vi "ElevatorControl.vi"(2 "Intake Active":bool, 3 "BallThereAtBottom?":bool, 4 "BallThereAtTop?":bool, 5 "WantToShoot?":bool) -> (0 "HopperWheelsOn":bool, 1 "ElevatorOn":bool)   [LabVIEW 2019]
uses:
  ArgosLib/ArgosLib.lvlib
panel:
  in  "IntakeHopperTime(ms)":u32=1000
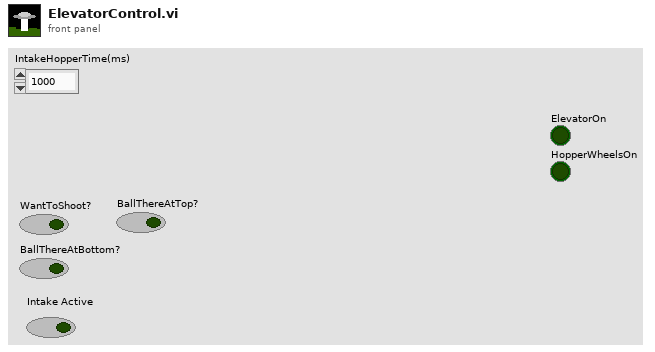
[diagram p1: front panel]
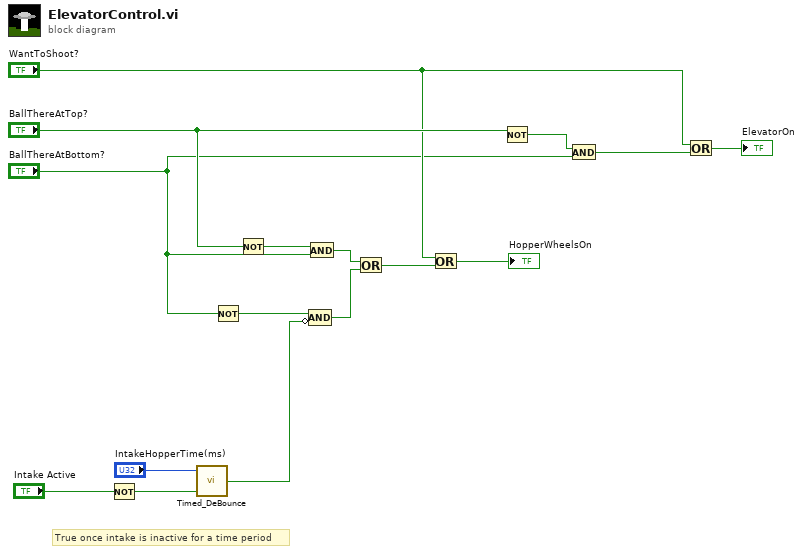
[diagram p0: block diagram]
diagram:
  # "True once intake is inactive for a time period"
  n1 = Not(x="Intake Active") -> (.not. x?=w7:bool)
  n2 = call "Timed_DeBounce.vi"("Input"=w7, "Hold Time(ms)"="IntakeHopperTime(ms)") -> ("Output"=w3:bool)  [unwired: 1 in]
  n3 = Not(x="BallThereAtBottom?") -> (.not. x?=w4:bool)
  n4 = Not(x="BallThereAtTop?") -> (.not. x?=w2:bool)
  n5 = And(x=w2, y="BallThereAtBottom?") -> (x .and. y?=w13:bool)
  n6 = Compound Arithmetic op=AND(w4, invert w3) -> (w5:bool)
  n7 = Or(x=w13, y=w5) -> (x .or. y?=w10:bool)
  n8 = Or(x="WantToShoot?", y=w10) -> (x .or. y?=→"HopperWheelsOn":bool)
  n9 = Not(x="BallThereAtTop?") -> (.not. x?=w16:bool)
  n10 = And(x=w16, y="BallThereAtBottom?") -> (x .and. y?=w15:bool)
  n11 = Or(x="WantToShoot?", y=w15) -> (x .or. y?=→"ElevatorOn":bool)
